vi "Format AK Response.vi"(8 "error in (no error)":errorcluster, 10 "Current Command Code":string, 11 "Response":string) -> (0 "error out":errorcluster, 3 "Data":string)   [LabVIEW 2013, in "Protocol Classes.lvlib"]
uses:
  Protocol Classes.lvlib
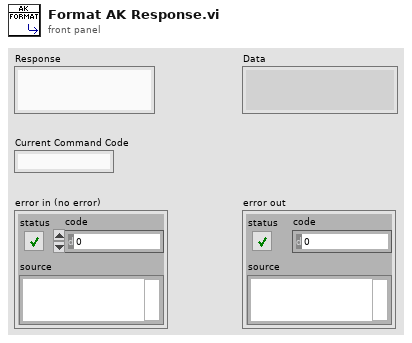
[diagram p1: front panel]
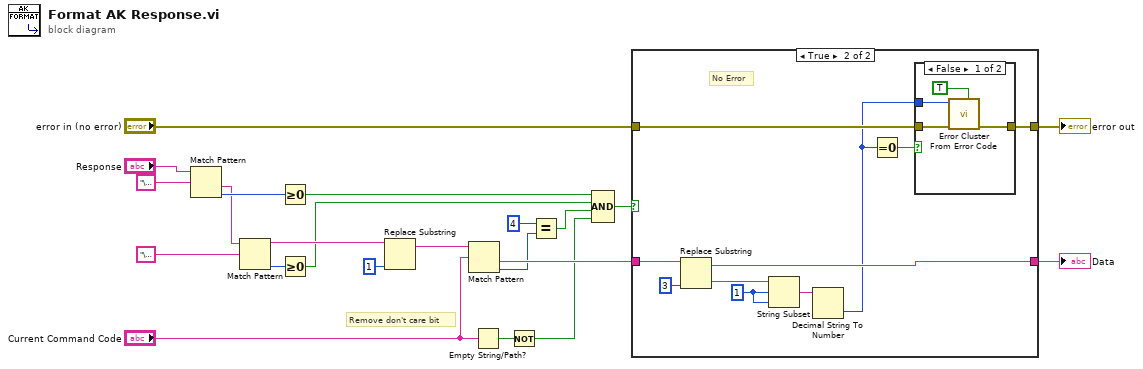
[diagram p0: block diagram]
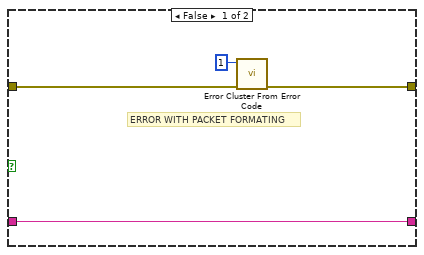
[diagram p2: hidden frame]
diagram:
  # "Remove don't care bit"
  n1 = Match Pattern(string="Response", regular expression="\u0002") -> (after substring=w6:string, offset past match=w9:i32)  [unwired: 1 in, 2 out]
  n2 = Match Pattern(string=w6, regular expression="\u0003") -> (before substring=w17:string, offset past match=w8:i32)  [unwired: 1 in, 2 out]
  n3 = Greater Or Equal To 0?(x=w9) -> (x >= 0?=w10:bool)
  n4 = Greater Or Equal To 0?(x=w8) -> (x >= 0?=w11:bool)
  n5 = Replace Substring(2:1 ("length (len. of substring)"), 5:w17) -> (1:w18:string)  [unwired: 2 in, 1 out]
  n6 = Match Pattern(string=w18, regular expression="Current Command Code") -> (after substring=w15:string, offset past match=w12:i32)  [unwired: 1 in, 2 out]
  n7 = Empty String/Path?(string/path="Current Command Code") -> (empty?=w2:bool)
  n8 = Not(x=w2) -> (.not. x?=w1:bool)
  n9 = Equal?(x=4, y=w12) -> (x = y?=w14:bool)
  n10 = Compound Arithmetic op=AND(w10, w11, w14, w1) -> (w20:bool)
  n11 = case shown="True" w20 {
    tunnel: w15 -> [w26 w35]
    tunnel: [w26 w34] -> w19
    tunnel: [w24 w29] -> w22
    tunnel: "error in (no error)" -> [w25 w30]
    frame False {
      # "ERROR WITH PACKET FORMATING"
      n12 = call <vilib>:"Error Cluster From Error Code.vi"("error in (no error)"=w25, "error code (0)"=1) -> ("error out"=w24:errorcluster)  [unwired: 7 in]
    }
    frame True {
      w33 = 1 ("offset (0)")
      # "No Error"
      n13 = Replace Substring(2:3 ("length (len. of substring)"), 5:w35) -> (0:w27:string, 1:w34:string)  [unwired: 2 in]
      n14 = String Subset(string=w27, offset (0)=w33, length (rest)=w33) -> (substring=w32:string)
      n15 = Decimal String To Number(string=w32) -> (number=w28:i32)  [unwired: 2 in, 1 out]
      n16 = Equal To 0?(x=w28) -> (x = 0?=w31:bool)
      n17 = case shown="False" w31 {
        tunnel: w30 -> [w40 w41]
        tunnel: [w39 w41] -> w29
        tunnel: w28 -> [w38 _]
        frame False {
          n18 = call <vilib>:"Error Cluster From Error Code.vi"("is warning? (False)"=TRUE, "error in (no error)"=w40, "error code (0)"=w38) -> ("error out"=w39:errorcluster)  [unwired: 6 in]
        }
        frame True {
          # "No Error"
        }
      }
    }
  }
  "error out" <- w22
  "Data" <- w19
